vi "InputSN_BMU.vi"(6 "TestCnt":dbl, 7 "目标板号":u8=1 max=30, 8 "CCM_Result":bool[](array[boolean]), 9 "BMU":string, 11 "Sequence Context In":refnum<k7>) -> (0 "error out":errorcluster, 1 "目标板号 2":u8=1 min=1 max=30, 2 "stop":bool=TRUE, 3 "Report Text":string, 10 "Boolean":bool)   [LabVIEW 2018]
panel:
  in  "CCM 5":string
  in  "CCM 4":string
  in  "CCM 3":string
  in  "CCM 2":string
  in  "CCM 1":string
  in  "请输入条码":string
  in  "STOP":bool
  in  "START":bool
  # "请输入/扫描条码&&目标板号"
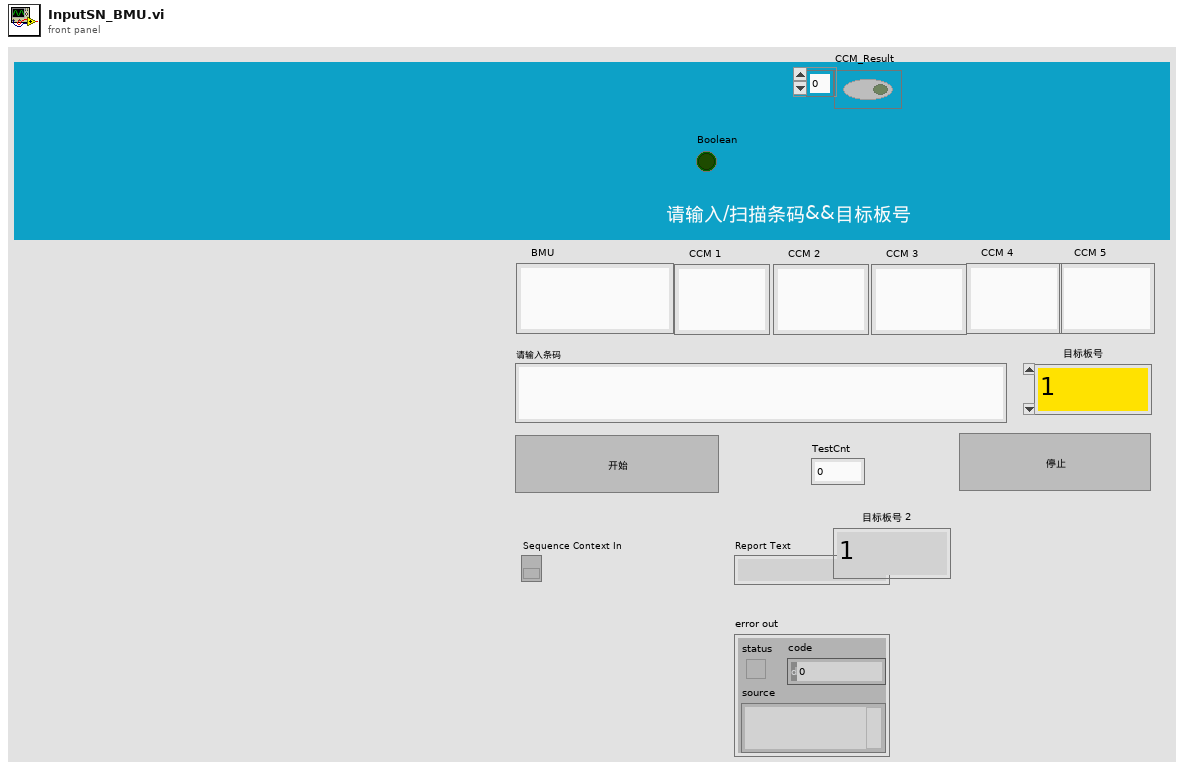
[diagram p1: front panel]
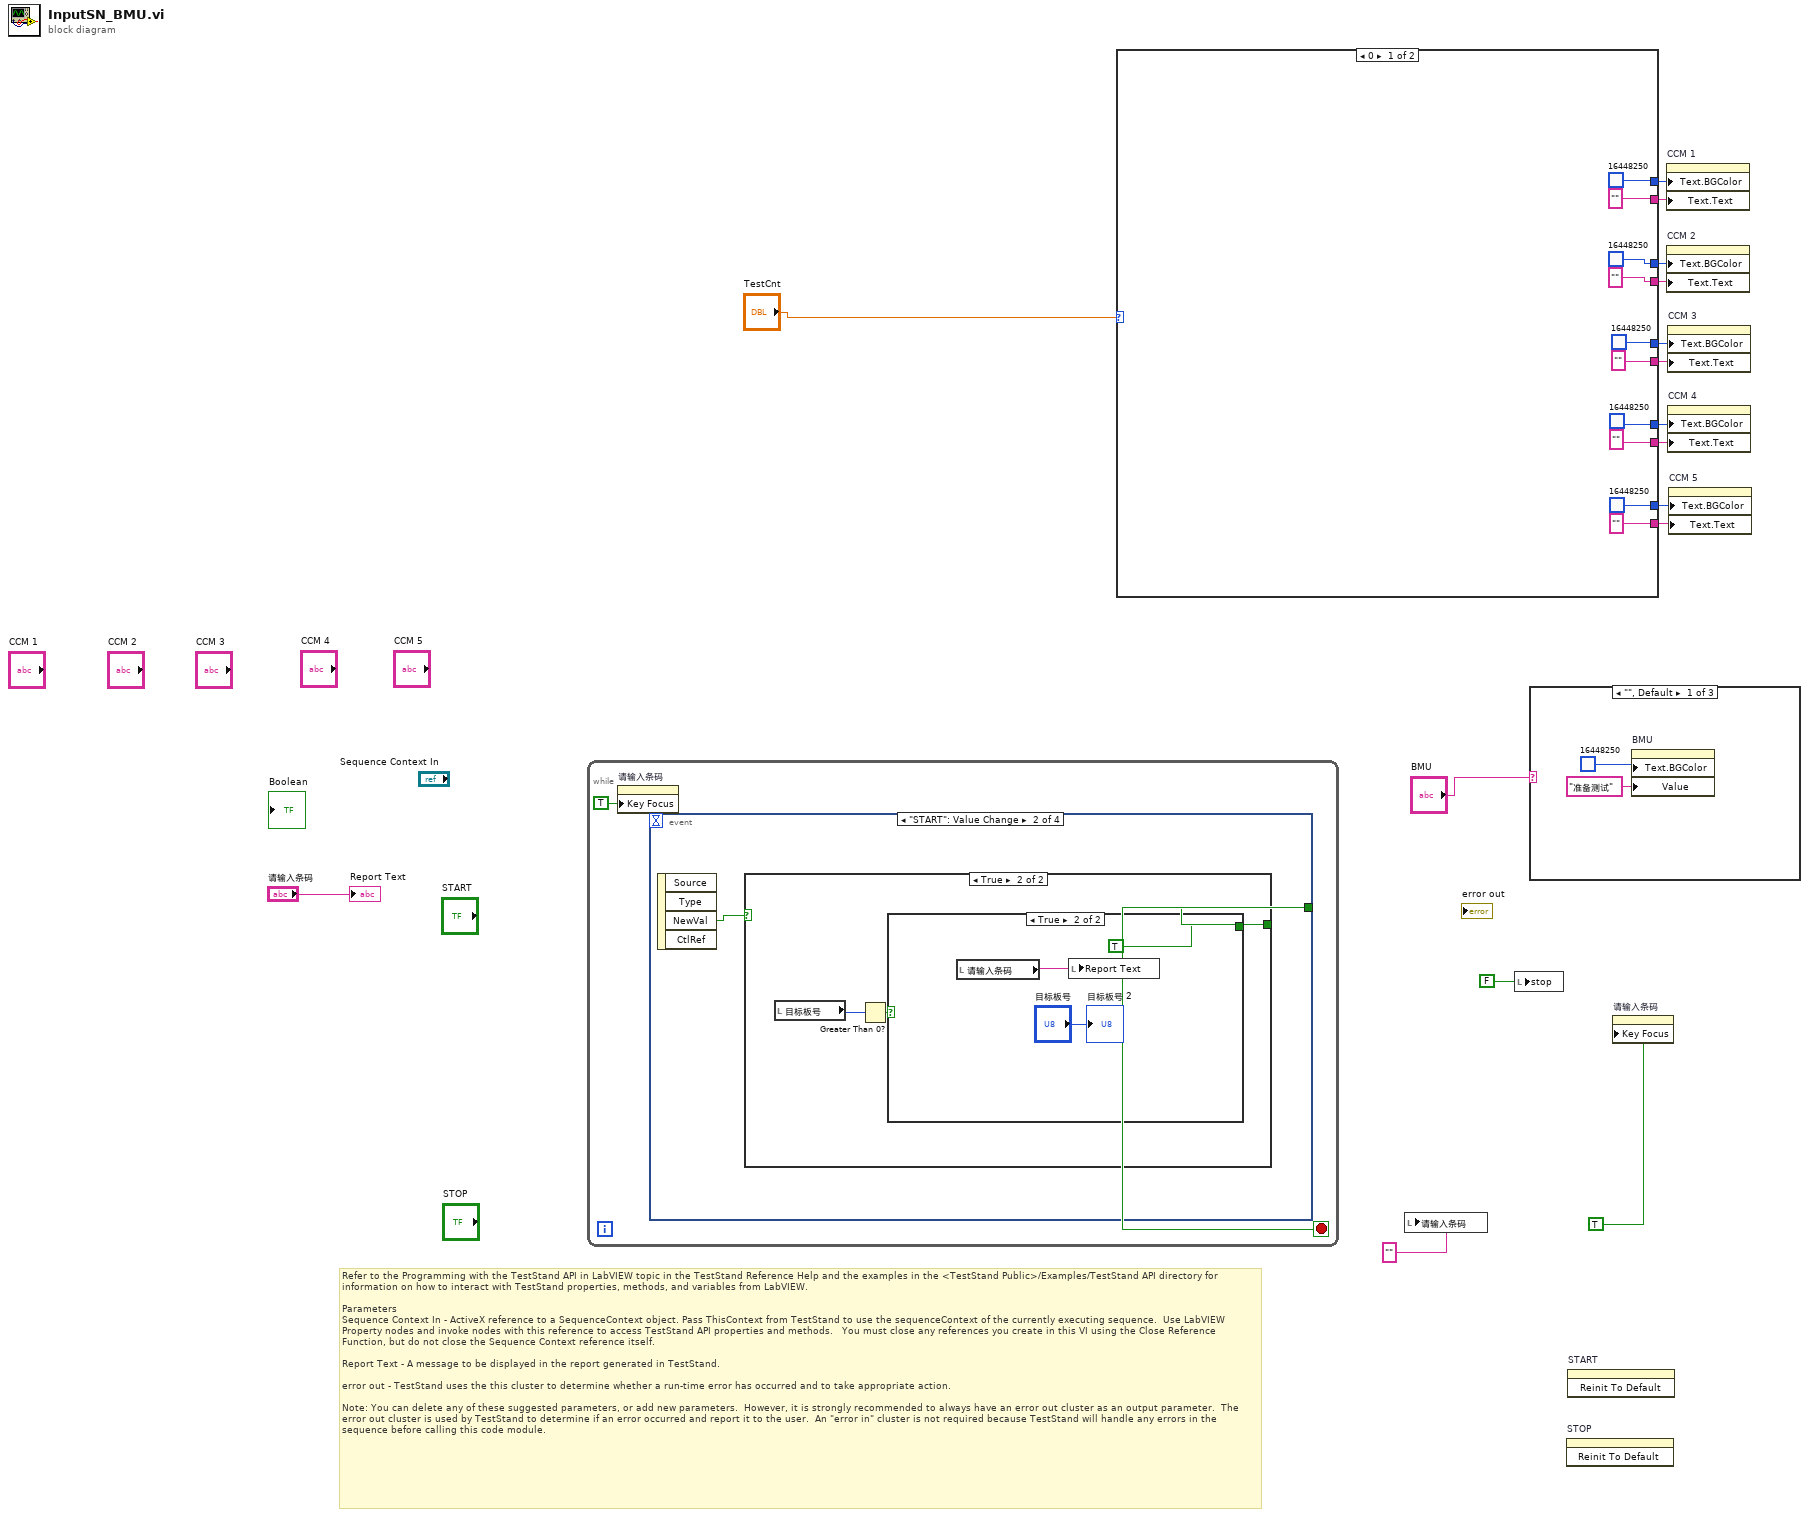
[diagram p0: block diagram]
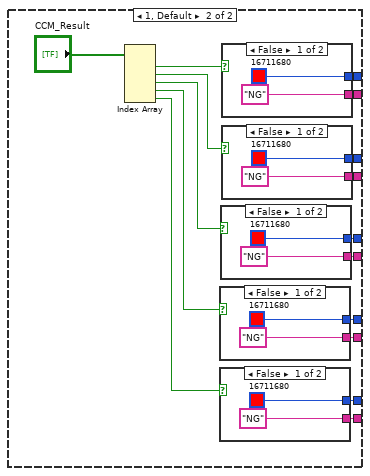
[diagram p2: hidden frame]
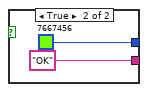
[diagram p3: hidden frame]
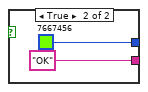
[diagram p4: hidden frame]
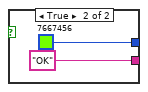
[diagram p5: hidden frame]
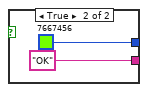
[diagram p6: hidden frame]
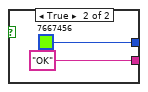
[diagram p7: hidden frame]
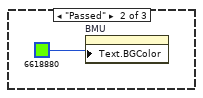
[diagram p8: hidden frame]
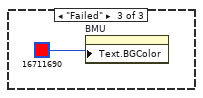
[diagram p9: hidden frame]
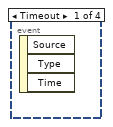
[diagram p10: hidden frame]
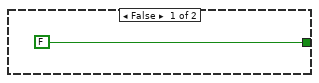
[diagram p11: hidden frame]
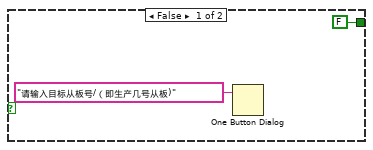
[diagram p12: hidden frame]
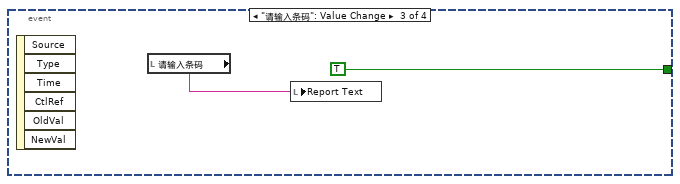
[diagram p13: hidden frame]
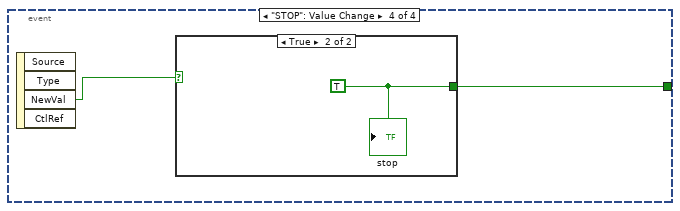
[diagram p14: hidden frame]
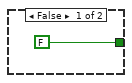
[diagram p15: hidden frame]
diagram:
  # "Refer to the Programming with the TestStand API in LabVIEW topic in the TestStand Reference Help and the examples in the <TestStand Public>/Examples/TestStand API directory for information on how to interact with TestStand properties, methods, and variables from LabVIEW.\n\nParameters\nSequence Context In - ActiveX reference to a SequenceContext object. Pass ThisContext from TestStand to use the sequenceContext of the currently executing sequence.  Use LabVIEW Property nodes and invoke nodes with this reference to access TestStand API properties and methods.   You must close any references you create in this VI using the Close Reference Function, but do not close the Sequence Context reference itself.\n\nReport Text - A message to be displayed in the report generated in TestStand. \n\nerror out - TestStand uses the this cluster to determine whether a run-time error has occurred and to take appropriate action.  \n\nNote: You can delete any of these suggested parameters, or add new parameters.  However, it is strongly recommended to always have an error out cluster as an output parameter.  The error out cluster is used by TestStand to determine if an error occurred and report it to the user.  An \"error in\" cluster is not required because TestStand will handle any errors in the sequence before calling this code module."
  n1 = while {
    stop <- w18 stop-if-true
    n2 = property on="请输入条码" class="Str"("Key Focus"=TRUE) -> ()  [unwired: 2 in, 2 out]
    n3 = event shown="[1] \"START\": Value Change" {
      selector: _ -> [_ _ _ _]
      dyn-events: _ -> [_ _ _ _]
      timeout: _ -> [_ _ _ _]
      tunnel: [_ w19 TRUE w32] -> w18
      event Timeout {
        n4 = event-data() -> ()  [unwired: 1 in, 3 out]
      }
      event "START": Value Change {
        n5 = event-data() -> ("NewVal"=w20:bool)  [unwired: 1 in, 3 out]
        n6 = case shown="True" w20 {
          tunnel: [FALSE w24] -> w19
          frame False {
          }
          frame True {
            n7 = local read "目标板号"() -> (w23:u8)
            n8 = Greater Than 0?(x=w23) -> (x > 0?=w22:bool)
            n9 = case shown="True" w22 {
              tunnel: [FALSE TRUE] -> w24
              frame False {
                n10 = One Button Dialog(message="请输入目标从板号/（即生产几号从板)") -> ()  [unwired: 1 in, 1 out]
              }
              frame True {
                n11 = local read "请输入条码"() -> (w28:string)
                n12 = local write "Report Text"(w28) -> ()
                "目标板号 2" <- "目标板号"
              }
            }
          }
        }
      }
      event "请输入条码": Value Change {
        n13 = event-data() -> ()  [unwired: 1 in, 6 out]
        n14 = local read "请输入条码"() -> (w30:string)
        n15 = local write "Report Text"(w30) -> ()
      }
      event "STOP": Value Change {
        n16 = event-data() -> ("NewVal"=w33:bool)  [unwired: 1 in, 3 out]
        n17 = case shown="True" w33 {
          tunnel: [FALSE w35] -> w32
          frame False {
          }
          frame True {
            w35 = TRUE
            "stop" <- w35
          }
        }
      }
    }
  }
  n18 = case shown="0" "TestCnt" {
    tunnel: [u32 16448250 w59] -> w11
    tunnel: ["" ("Text.Text") w58] -> w10
    tunnel: ["" ("Text.Text") w57] -> w9
    tunnel: ["" ("Text.Text") w56] -> w8
    tunnel: ["" ("Text.Text") w55] -> w7
    tunnel: [u32 16448250 w50] -> w6
    tunnel: [u32 16448250 w49] -> w5
    tunnel: ["" ("Text.Text") w48] -> w4
    tunnel: [u32 16448250 w47] -> w3
    tunnel: [u32 16448250 w46] -> w2
    frame 0 {
    }
    frame 1, Default {
      n19 = Index Array(array="CCM_Result") -> (element #1=w60:bool, element #2=w54:bool, element #3=w53:bool, element #4=w52:bool, element #5=w51:bool)  [unwired: 5 in]
      n20 = case shown="False" w52 {
        tunnel: [u32 16711680 u32 7667456] -> w49
        tunnel: ["NG" ("Text.Text") "OK" ("Text.Text")] -> w48
        frame False {
        }
        frame True {
        }
      }
      n21 = case shown="False" w51 {
        tunnel: [u32 16711680 u32 7667456] -> w50
        tunnel: ["NG" ("Text.Text") "OK" ("Text.Text")] -> w55
        frame False {
        }
        frame True {
        }
      }
      n22 = case shown="False" w53 {
        tunnel: [u32 16711680 u32 7667456] -> w47
        tunnel: ["NG" ("Text.Text") "OK" ("Text.Text")] -> w56
        frame False {
        }
        frame True {
        }
      }
      n23 = case shown="False" w60 {
        tunnel: [u32 16711680 u32 7667456] -> w59
        tunnel: ["NG" ("Text.Text") "OK" ("Text.Text")] -> w58
        frame False {
        }
        frame True {
        }
      }
      n24 = case shown="False" w54 {
        tunnel: [u32 16711680 u32 7667456] -> w46
        tunnel: ["NG" ("Text.Text") "OK" ("Text.Text")] -> w57
        frame False {
        }
        frame True {
        }
      }
    }
  }
  n25 = local write "请输入条码"("" ("请输入条码")) -> ()
  n26 = local write "stop"(FALSE ("Boolean")) -> ()
  n27 = case shown="\"\", Default" "BMU" {
    frame "", Default {
      n28 = property on="BMU" class="Str"("Text.BGColor"=u32 16448250, "Value"="准备测试" ("上一次测试结果")) -> ()  [unwired: 2 in, 2 out]
    }
    frame "Passed" {
      n29 = property on="BMU" class="Str"("Text.BGColor"=u32 6618880) -> ()  [unwired: 2 in, 2 out]
    }
    frame "Failed" {
      n30 = property on="BMU" class="Str"("Text.BGColor"=u32 16711690) -> ()  [unwired: 2 in, 2 out]
    }
  }
  n31 = invoke on="STOP" class="Bool (strict)" method="Reinit To Default"() -> ()  [unwired: 3 in, 3 out]
  n32 = invoke on="START" class="Bool (strict)" method="Reinit To Default"() -> ()  [unwired: 3 in, 3 out]
  n33 = property on="请输入条码" class="Str"("Key Focus"=TRUE) -> ()  [unwired: 2 in, 2 out]
  n34 = property on="CCM 1" class="Str"("Text.BGColor"=w11, "Text.Text"=w10) -> ()  [unwired: 2 in, 2 out]
  n35 = property on="CCM 2" class="Str"("Text.BGColor"=w2, "Text.Text"=w9) -> ()  [unwired: 2 in, 2 out]
  n36 = property on="CCM 3" class="Str"("Text.BGColor"=w3, "Text.Text"=w8) -> ()  [unwired: 2 in, 2 out]
  n37 = property on="CCM 4" class="Str"("Text.BGColor"=w5, "Text.Text"=w4) -> ()  [unwired: 2 in, 2 out]
  n38 = property on="CCM 5" class="Str"("Text.BGColor"=w6, "Text.Text"=w7) -> ()  [unwired: 2 in, 2 out]
  "Report Text" <- "请输入条码"
